vi "Vision Server Clear Vision Updates.vi"(1 "Vision Server":T1={"connection ID"=refnum, "Running?"=TRUE, "TCP Port"=65535, "LastMessageReceivedTime"=0.0, "WantsAppRestart"=FALSE, "IsConnect"=FALSE, "Targets Updates"=[{"Valid?"=FALSE, "CapturedAtTimestamp"=0.0, "Targets Message"={"capturedAgoMs"=0, "targets"=[{"x"=0.0, "y"=0.0, "z"=0.0, "theta"=0.0}]}}]}) -> (0 "Vision Server":T1={"connection ID"=refnum, "Running?"=TRUE, "TCP Port"=65535, "LastMessageReceivedTime"=0.0, "WantsAppRestart"=FALSE, "IsConnect"=FALSE, "Targets Updates"=[{"Valid?"=FALSE, "CapturedAtTimestamp"=0.0, "Targets Message"={"capturedAgoMs"=0, "targets"=[{"x"=0.0, "y"=0.0, "z"=0.0, "theta"=0.0}]}}]})   [LabVIEW 2016]
uses:
  Vision Server.ctl
  Messages/Targets/Targets Update.ctl
  Messages/Targets/Targets Message.ctl
  Messages/Targets/Targets Info.ctl
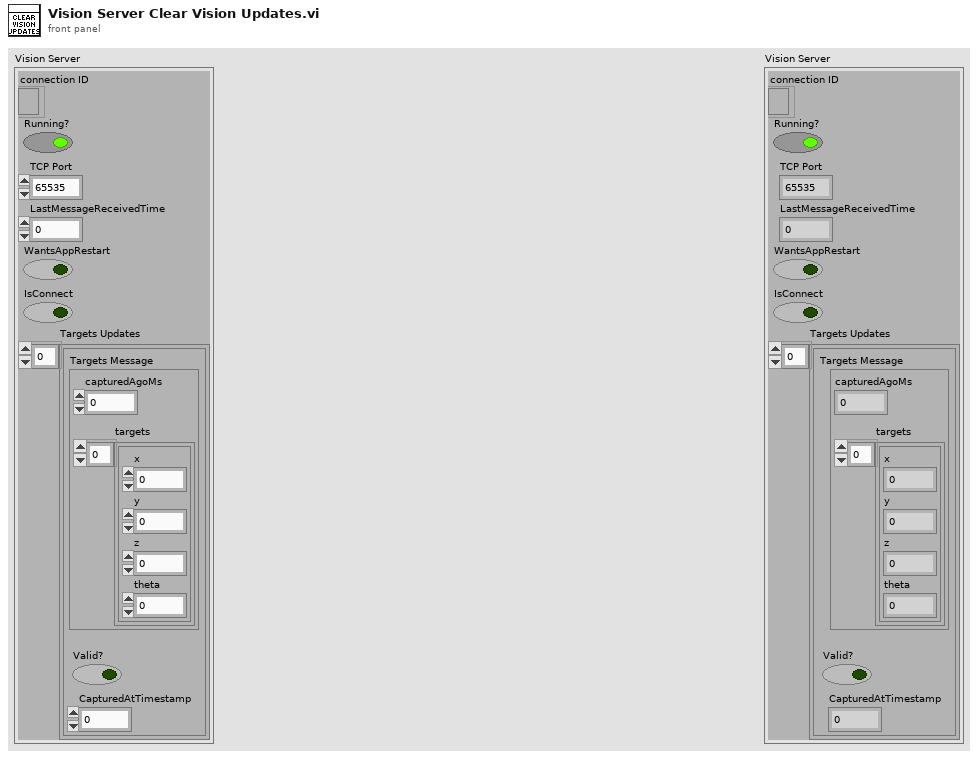
[diagram p1: front panel]
types:
  T1 = typedef "Vision Server.ctl" = cluster{"connection ID":refnum<k5>, "Running?":bool, "TCP Port":u16, "LastMessageReceivedTime":dbl, "WantsAppRestart":bool, "IsConnect":bool, "Targets Updates":T2[]}
  T2 = typedef "Targets Update.ctl" = cluster{"Valid?":bool, "CapturedAtTimestamp":dbl, "Targets Message":T3}
  T3 = typedef "Targets Message.ctl" = cluster{"capturedAgoMs":i32, "targets":T4[]}
  T4 = typedef "Targets Info.ctl" = cluster{"x":dbl, "y":dbl, "z":dbl, "theta":dbl}
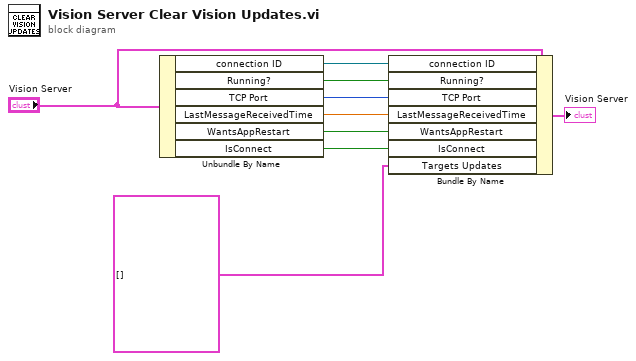
[diagram p0: block diagram]
diagram:
  n1 = Unbundle By Name("Vision Server") -> ("connection ID"=w9:refnum<k5>, "Running?"=w8:bool, "TCP Port"=w7:u16, "LastMessageReceivedTime"=w6:dbl, "WantsAppRestart"=w5:bool, "IsConnect"=w4:bool)
  n2 = Bundle By Name(cluster="Vision Server", "connection ID"=w9, "Running?"=w8, "TCP Port"=w7, "LastMessageReceivedTime"=w6, "WantsAppRestart"=w5, "IsConnect"=w4, "Targets Updates"=T2[] []) -> (→"Vision Server":T1)
